vi "maze_v9.vi"   [LabVIEW 2012]
uses:
  <vilib>/NXT/Subs/MotorOutput.ctl
  <vilib>/NXT/Block Support/NXT_InputPort.ctl
  <vilib>/NXT/Dual Mode Library/Motors/MotorBrake.vi
  <vilib>/NXT/Dual Mode Library/prims/addArrayElements_int.vi
  <vilib>/NXT/Dual Mode Library/Motors/MotorOn.vi
  <vilib>/NXT/Dual Mode Library/Waits/Wait_Num(msec).vi
types:
  T1 = typedef "MotorOutput.ctl" = u8
  T2 = typedef "LVHSConnector.ctl" = cluster{"Hardware":string, "Flattened String":string}
  T3 = typedef "NXT_InputPort.ctl" = u8
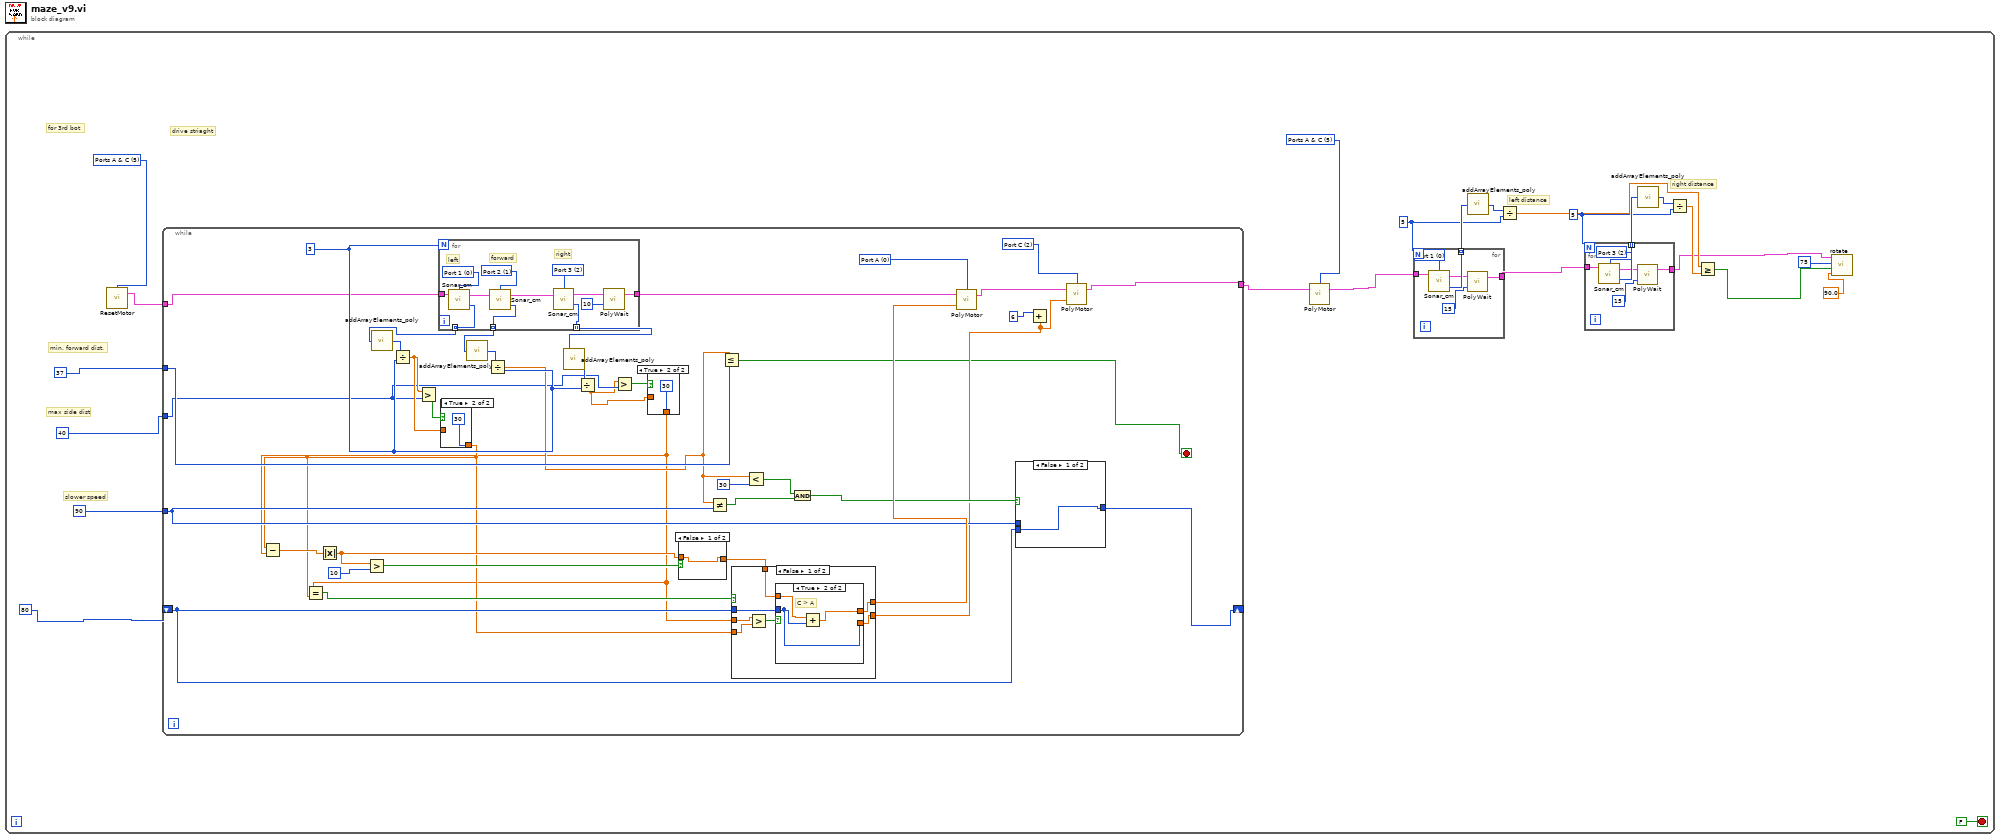
[diagram p0: block diagram]
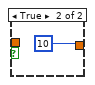
[diagram p4: hidden frame]
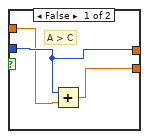
[diagram p6: hidden frame]
diagram:
  n1 = while {
    stop <- FALSE stop-if-true
    w7 = 5
    w10 = 5
    w23 = T1 5 items=["Port A"=0, "Port B"=1, "Port C"=2, "Ports A & B"=4, "Ports A & C"=5, "Ports B & C"=6, "All Ports"=3] ("Output Port (All Ports)")
    w21 = T1 5 items=["Port A"=0, "Port B"=1, "Port C"=2, "Ports A & B"=4, "Ports A & C"=5, "Ports B & C"=6, "All Ports"=3] ("Output Port (All Ports)")
    # "right distance"
    # "left distance"
    # "max side dist"
    # "drive striaght"
    # "for 3rd bot"
    # "min. forward dist."
    # "slower speed"
    n2 = call <vilib>:"ResetMotor.vi"("Port (All Ports)"=w21) -> ("NXT"=w22:T2)  [unwired: 3 in]
    n3 = while {
      tunnel: w22 -> [w46]
      tunnel: [w36] -> w20
      tunnel: 37 -> [w69]
      shift-right: [w63] -> _
      shift-left: 80 -> [w62]
      tunnel: 90 -> [w53]
      tunnel: 40 -> [w40]
      stop <- w37 stop-if-true
      w48 = 3
      w72 = T1 2 items=["Port A"=0, "Port B"=1, "Port C"=2, "Ports A & B"=4, "Ports A & C"=5, "Ports B & C"=6, "All Ports"=3] ("Output Port (All Ports)")
      w73 = T1 0 items=["Port A"=0, "Port B"=1, "Port C"=2, "Ports A & B"=4, "Ports A & C"=5, "Ports B & C"=6, "All Ports"=3] ("Output Port (All Ports)")
      n4 = for {
        N: w48 -> [_]
        tunnel: w46 -> [w85]
        tunnel: [w88] -> w70
        tunnel: [w89] -> w55 mode=indexing
        tunnel: [w80] -> w52 mode=indexing
        tunnel: [w79] -> w51 mode=indexing
        w81 = T3 1 items=["Port 1", "Port 2", "Port 3", "Port 4"] ("Port (Port 4)")
        w82 = T3 0 items=["Port 1", "Port 2", "Port 3", "Port 4"] ("Port (Port 4)")
        w90 = T3 2 items=["Port 1", "Port 2", "Port 3", "Port 4"] ("Port (Port 4)")
        # "right"
        # "forward"
        # "left"
        n5 = call <vilib>:"Sonar_cm.vi"("NXT"=w85, "Port (Port 4)"=w82) -> ("Distance (cm)"=w80:i16, "NXT"=w84:T2)  [unwired: 1 in]
        n6 = call <vilib>:"Sonar_cm.vi"("NXT"=w84, "Port (Port 4)"=w81) -> ("Distance (cm)"=w79:i16, "NXT"=w83:T2)  [unwired: 1 in]
        n7 = call <vilib>:"Sonar_cm.vi"("NXT"=w83, "Port (Port 4)"=w90) -> ("Distance (cm)"=w89:i16, "NXT"=w87:T2)  [unwired: 1 in]
        n8 = call-poly <vilib>:"PolyWait.vi"("Time (100 msec)"=10, "NXT"=w87) -> ("NXT"=w88:T2)  [unwired: 2 in]
      }
      n9 = call-poly <vilib>:"addArrayElements_poly.vi"("Numeric Array"=w52) -> ("Sum"=w49:i32)
      n10 = Divide(x=w49, y=w48) -> (x/y=w44:dbl)
      n11 = Greater?(x=w44, y=w40) -> (0:w45:bool)
      n12 = case shown="True" w45 {
        tunnel: [w77 30] -> w43
        tunnel: w44 -> [w77 _]
        frame False {
        }
        frame True {
        }
      }
      n13 = call-poly <vilib>:"addArrayElements_poly.vi"("Numeric Array"=w51) -> ("Sum"=w50:i32)
      n14 = Divide(x=w50, y=w48) -> (x/y=w42:dbl)
      n15 = call-poly <vilib>:"addArrayElements_poly.vi"("Numeric Array"=w55) -> ("Sum"=w54:i32)
      n16 = Divide(x=w54, y=w48) -> (x/y=w39:dbl)
      n17 = Greater?(x=w39, y=w40) -> (0:w41:bool)
      n18 = case shown="True" w41 {
        tunnel: [w75 30] -> w38
        tunnel: w39 -> [w75 _]
        frame False {
        }
        frame True {
        }
      }
      n19 = Subtract(x=w43, y=w38) -> (x-y=w61:dbl)
      n20 = Equal?(x=w38, y=w43) -> (x = y?=w71:bool)
      n21 = Absolute Value(x=w61) -> (abs(x)=w58:dbl)
      n22 = Greater?(x=w58, y=10) -> (0:w59:bool)
      n23 = case shown="False" w59 {
        tunnel: [w91 10] -> w57
        tunnel: w58 -> [w91 _]
        frame False {
        }
        frame True {
        }
      }
      n24 = Not Equal?(x=w42, y=w53) -> (x != y?=w65:bool)
      n25 = Less Or Equal?(x=w42, y=w69) -> (x <= y?=w37:bool)
      n26 = case shown="False" w71 {
        tunnel: [w99 w108] -> w68
        tunnel: w62 -> [w100 w108]
        tunnel: [w98 w108] -> w47
        tunnel: w43 -> [w97 _]
        tunnel: w38 -> [w96 _]
        tunnel: w57 -> [w95 _]
        frame False {
          n27 = Greater?(x=w96, y=w97) -> (0:w101:bool)
          n28 = case shown="True" w101 {
            tunnel: w100 -> [w103 w107]
            tunnel: [w103 w105] -> w99
            tunnel: [w104 w107] -> w98
            tunnel: w95 -> [w102 w106]
            frame False {
              # "A > C"
              n29 = Add(x=w103, y=w102) -> (x+y=w104:dbl)
            }
            frame True {
              # "C > A"
              n30 = Add(x=w106, y=w107) -> (x+y=w105:dbl)
            }
          }
        }
        frame True {
        }
      }
      n31 = Less?(x=w42, y=30) -> (x < y?=w66:bool)
      n32 = And(x=w66, y=w65) -> (x .and. y?=w64:bool)
      n33 = call-poly <vilib>:"PolyMotor.vi"("Power (75)"=w68, "NXT"=w70, "Output Port (All Ports)"=w73) -> ("NXT"=w74:T2)  [unwired: 1 in]
      n34 = case shown="False" w64 {
        tunnel: [w93 w94] -> w63
        tunnel: w62 -> [w93 _]
        tunnel: w53 -> [_ w94]
        frame False {
        }
        frame True {
        }
      }
      n35 = Add(x=6, y=w47) -> ()  [unwired: 1 out]
      n36 = call-poly <vilib>:"PolyMotor.vi"("Power (75)"=w47, "NXT"=w74, "Output Port (All Ports)"=w72) -> ("NXT"=w36:T2)  [unwired: 1 in]
    }
    n37 = call-poly <vilib>:"PolyMotor.vi"("NXT"=w20, "Port (All Ports)"=w23) -> ("NXT"=w2:T2)  [unwired: 2 in]
    n38 = for {
      N: w10 -> [_]
      tunnel: w2 -> [w34]
      tunnel: [w35] -> w12 mode=indexing
      tunnel: [w32] -> w6
      w30 = T3 0 items=["Port 1", "Port 2", "Port 3", "Port 4"] ("Port (Port 4)")
      n39 = call <vilib>:"Sonar_cm.vi"("NXT"=w34, "Port (Port 4)"=w30) -> ("Distance (cm)"=w35:i16, "NXT"=w33:T2)  [unwired: 1 in]
      n40 = call-poly <vilib>:"PolyWait.vi"("Time (100 msec)"=15, "NXT"=w33) -> ("NXT"=w32:T2)  [unwired: 2 in]
    }
    n41 = call-poly <vilib>:"addArrayElements_poly.vi"("Numeric Array"=w12) -> ("Sum"=w11:i32)
    n42 = Divide(x=w11, y=w10) -> (x/y=w5:dbl)
    n43 = for {
      N: w7 -> [_]
      tunnel: w6 -> [w28]
      tunnel: [w29] -> w9 mode=indexing
      tunnel: [w26] -> w1
      w24 = T3 2 items=["Port 1", "Port 2", "Port 3", "Port 4"] ("Port (Port 4)")
      n44 = call <vilib>:"Sonar_cm.vi"("NXT"=w28, "Port (Port 4)"=w24) -> ("Distance (cm)"=w29:i16, "NXT"=w27:T2)  [unwired: 1 in]
      n45 = call-poly <vilib>:"PolyWait.vi"("Time (100 msec)"=15, "NXT"=w27) -> ("NXT"=w26:T2)  [unwired: 2 in]
    }
    n46 = call-poly <vilib>:"addArrayElements_poly.vi"("Numeric Array"=w9) -> ("Sum"=w8:i32)
    n47 = Divide(x=w8, y=w7) -> (x/y=w4:dbl)
    n48 = Greater Or Equal?(x=w5, y=w4) -> (x >= y?=w13:bool)
    n49 = call "rotate.vi"("degrees to  rotate"=90.0, "right(T)/left(F)"=w13, "power"=u16 75, "NXT 2"=w1) -> ()  [unwired: 7 in, 1 out]
  }
